vi "z1.vi"() -> ()   [LabVIEW 2023]
panel:
  out "XY Graph":cluster{"X":dbl, "Y":dbl}[](graph)
  out "Waveform Chart":dbl(graph)
  out "Waveform Graph 3":dbl[](graph)
  out "Waveform Graph 2":dynamicdata(graph)
  out "Waveform Graph":dynamicdata(graph)
  out "Boolean 3":bool
  out "Boolean 2":bool
  in  "Boolean":bool
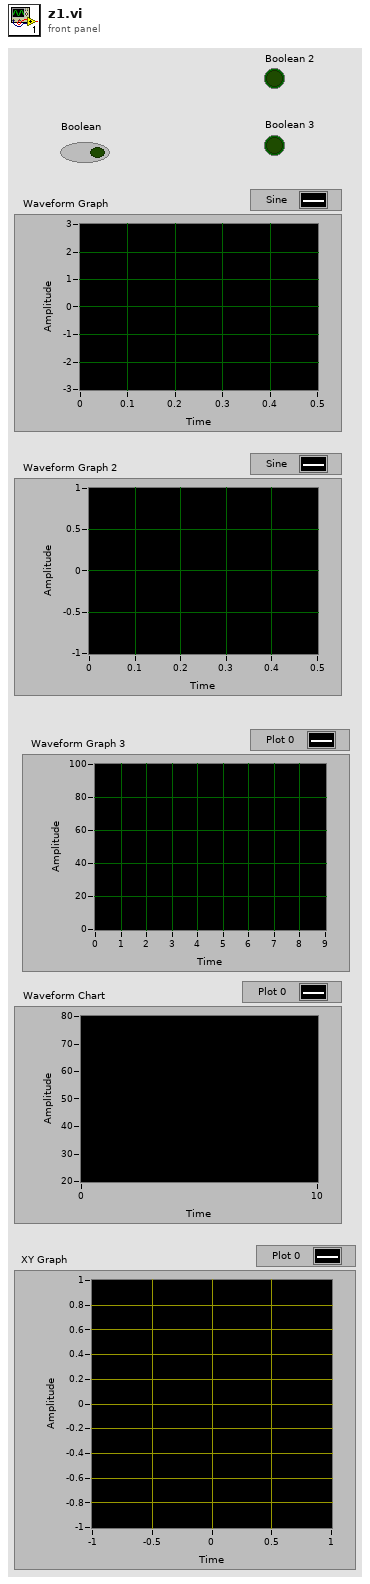
[diagram p1: front panel]
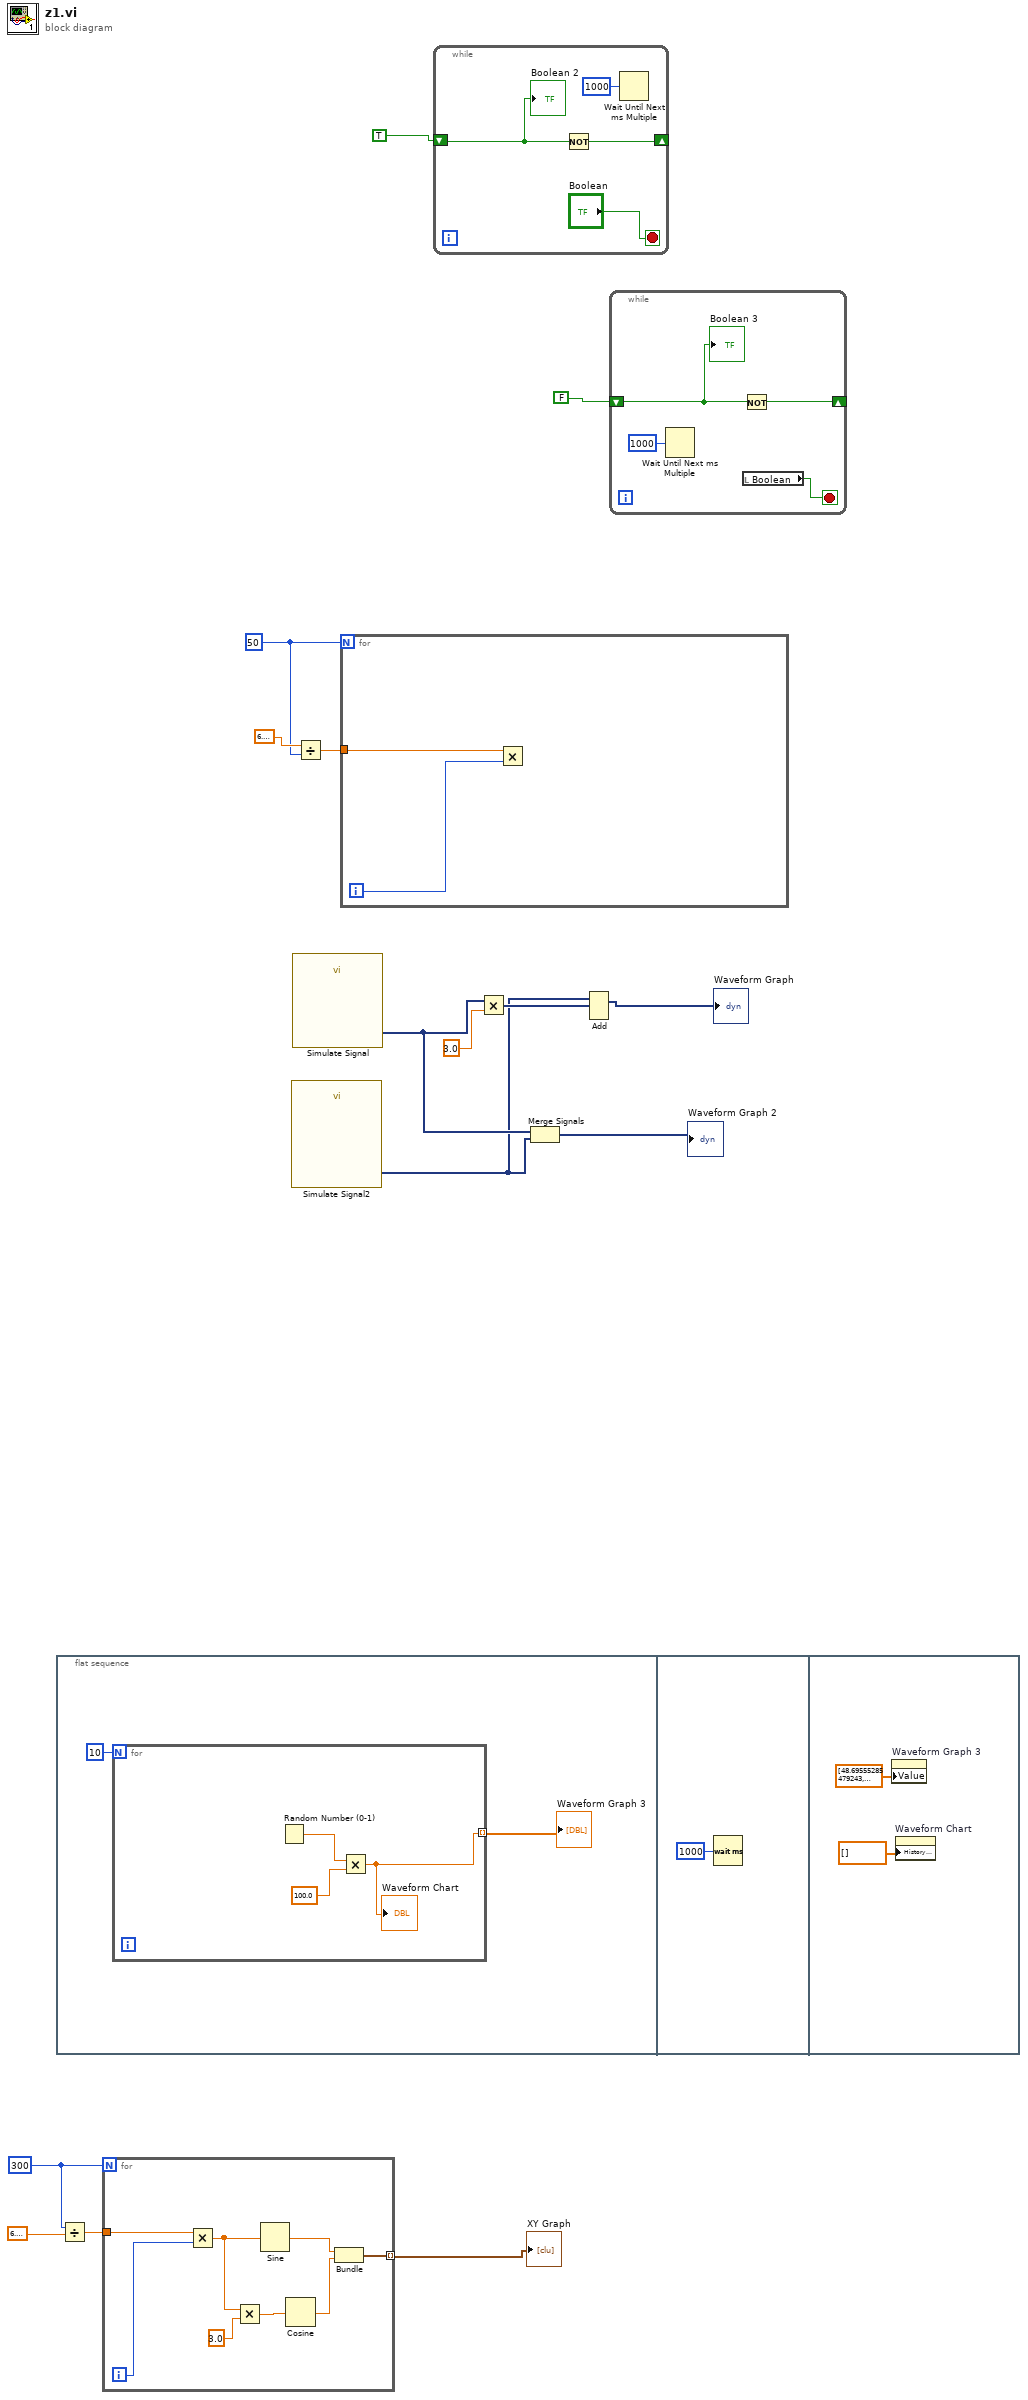
[diagram p0: block diagram]
diagram:
  w3 = 300
  w11 = 50
  n1 = flat-sequence {
    frame #0 {
      n2 = for {
        N: 10 -> [_]
        tunnel: [w18] -> w17 mode=indexing
        n3 = Random Number (0-1)() -> (number: 0 to 1=w19:dbl)
        n4 = Multiply(x=w19, y=100.0) -> (x*y=w18:dbl)
        "Waveform Chart" <- w18
      }
      "Waveform Graph 3" <- w17
    }
    frame #1 {
      n5 = Wait (ms)(milliseconds to wait=u32 1000) -> ()  [unwired: 1 out]
    }
    frame #2 {
      n6 = property on="Waveform Graph 3" class="WFGraph (strict)"("Value"=dbl[] [48.69555285479243, 77.84340433745291, 47.12111658936679, 6.113596640080532, 13.109062001003192, 95.8158429174384, 28.134832899330675, 10.1643698024793, 17.731022300516173, 47.056596335429916] ("Waveform Graph 3")) -> ()  [unwired: 2 in, 2 out]
      n7 = property on="Waveform Chart" class="WFChart (strict)"("History Data"=dbl[] []) -> ()  [unwired: 2 in, 2 out]
    }
  }
  n8 = Divide(x=w3, y=6.283185307179586) -> (x/y=w2:dbl)
  n9 = for {
    N: w3 -> [_]
    tunnel: w2 -> [w31]
    tunnel: [w26] -> w1 mode=indexing
    i -> [w30]
    n10 = Multiply(x=w31, y=w30) -> (x*y=w29:dbl)
    n11 = Multiply(x=w29, y=3.0) -> (x*y=w27:dbl)
    n12 = Sine(x=w29) -> (sin(x)=w25:dbl)
    n13 = Cosine(x=w27) -> (cos(x)=w24:dbl)
    n14 = Bundle(w25, w24) -> (w26:cluster{dbl, dbl})  [unwired: 1 in]
  }
  "XY Graph" <- w1
  n15 = call "Simulate Signal2"() -> ("Sine"=w6:dynamicdata)  [unwired: 14 in, 1 out]
  n16 = call "Simulate Signal"() -> ("Sine"=w9:dynamicdata)  [unwired: 14 in, 1 out]
  n17 = Divide(x=6.283185307179586, y=w11) -> (x/y=w12:dbl)
  n18 = for {
    N: w11 -> [_]
    tunnel: w12 -> [w32]
    i -> [w33]
    n19 = Multiply(x=w32, y=w33) -> ()  [unwired: 1 out]
  }
  n20 = while {
    shift-right: [w36] -> _
    shift-left: TRUE -> [w34]
    stop <- "Boolean" stop-if-true
    n21 = Not(x=w34) -> (.not. x?=w36:bool)
    n22 = Wait Until Next ms Multiple(millisecond multiple=u32 1000) -> ()  [unwired: 1 out]
    "Boolean 2" <- w34
  }
  n23 = Multiply(x=w9, y=3.0) -> (x*y=w7:dynamicdata)
  n24 = Merge Signals(w9, w6) -> (→"Waveform Graph 2":dynamicdata)
  n25 = Add(1:w7, 2:w6) -> (0:→"Waveform Graph":dynamicdata)  [unwired: 1 in, 1 out]
  n26 = while {
    shift-right: [w40] -> _
    shift-left: FALSE -> [w38]
    stop <- w41 stop-if-true
    n27 = Wait Until Next ms Multiple(millisecond multiple=u32 1000) -> ()  [unwired: 1 out]
    n28 = Not(x=w38) -> (.not. x?=w40:bool)
    n29 = local read "Boolean"() -> (w41:bool)
    "Boolean 3" <- w38
  }
